vi "RK_Ausgabe(SubVI).vi"(9 "Name":string, 11 "werS":string) -> (1 "AnzeigeBegrüß":string, 3 "AnzeigeOben":string)   [LabVIEW 2017]
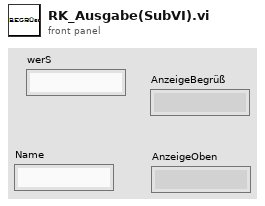
[diagram p1: front panel]
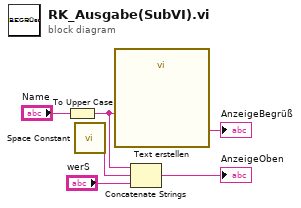
[diagram p0: block diagram]
diagram:
  n1 = To Upper Case(1:"Name") -> (0:w3:string)
  n2 = call <vilib>:"Space Constant.vi"() -> ("String"=w1:string)
  n3 = call "Text erstellen"("Name"=w3) -> ("Result"=→"AnzeigeBegrüß":string)  [unwired: 13 in, 1 out]
  n4 = Concatenate Strings(w3, w1, "werS") -> (→"AnzeigeOben":string)
